vi "Swap King Output String.vi"(0 "New Cell Index":i32, 5 "Old Cell Index":i32, 7 "Zero Indexed? (T)":bool=TRUE, 11 "error in (no error)":errorcluster) -> (4 "Output Text":string, 15 "error out":errorcluster)   [LabVIEW 2014]
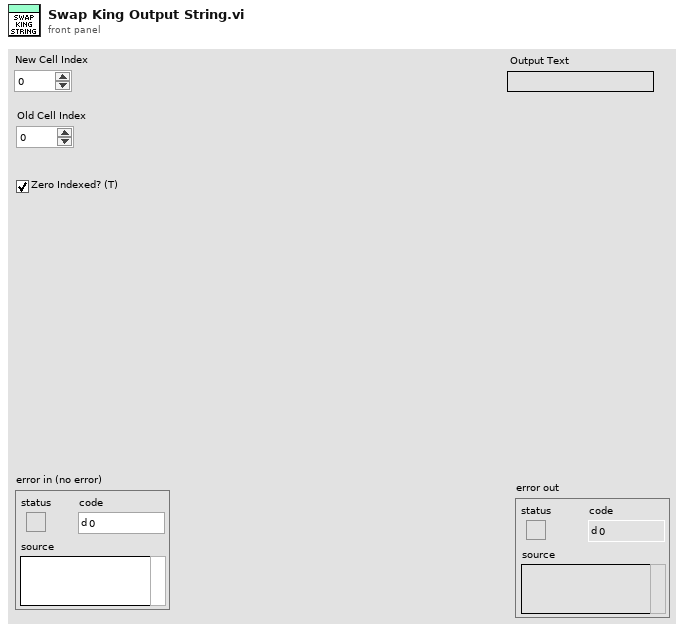
[diagram p1: front panel]
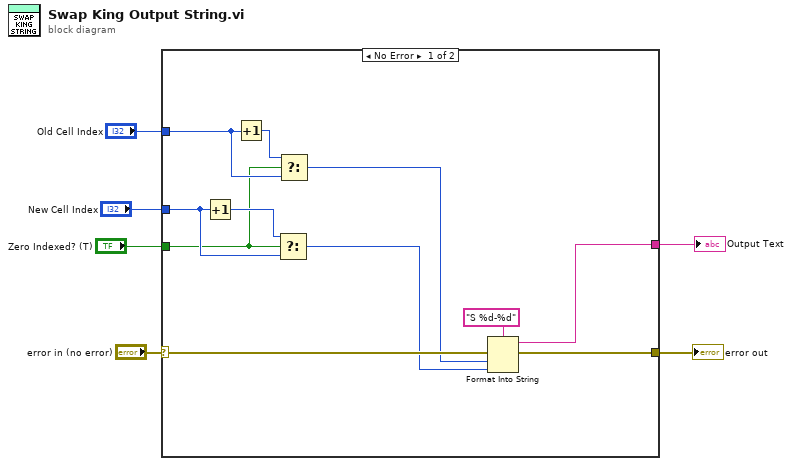
[diagram p0: block diagram]
diagram:
  n1 = case shown="No Error" "error in (no error)" {
    selector: "error in (no error)" -> [w16 w18]
    tunnel: [w15 w18] -> w5
    tunnel: "New Cell Index" -> [w12 _]
    tunnel: [w14 _] -> w3
    tunnel: "Zero Indexed? (T)" -> [w9 _]
    tunnel: "Old Cell Index" -> [w10 _]
    frame No Error {
      n2 = Increment(x=w12) -> (x+1=w13:i32)
      n3 = Increment(x=w10) -> (x+1=w11:i32)
      n4 = Select(t=w13, s=w9, f=w12) -> (s? t:f=w7:i32)
      n5 = Select(t=w11, s=w9, f=w10) -> (s? t:f=w8:i32)
      n6 = Format Into String(format string="S %d-%d", error in=w16, w8, w7) -> (resulting string=w14:string, error out=w15:errorcluster)  [unwired: 1 in]
    }
    frame Error {
    }
  }
  "error out" <- w5
  "Output Text" <- w3
